vi "GetProperty.vi"(7 "Get":bool, 8 "error in (no error)":errorcluster, 9 "SubIndex":u8 format="%x", 10 "Index":u16 format="%x", 11 "Template SoftMotion Drive Interface Plug-in Class in":refnum<class "Template SoftMotion Drive Interface Plug-in Class.lvclass">) -> (0 "error out":errorcluster, 1 "Data":u32, 2 "Done":bool, 3 "Template SoftMotion Drive Interface Plug-in Class out":refnum<class "Template SoftMotion Drive Interface Plug-in Class.lvclass">)   [LabVIEW 2014, in "Template SoftMotion Drive Interface Plug-in Class.lvclass"]
uses:
  Template SoftMotion Drive Interface Plug-in Class.lvclass
  <vilib>/Motion/plugins/PluginFramework/nismPluginAxisBase/nismPluginAxisBaseClass.lvclass/nismPluginAxisBaseClass.ctl
  <vilib>/Motion/plugins/PluginFramework/nismPluginAxisBase/ReadEtherCATSlaveReference.vi
  <resource>/objmgr/IndComECAT.rc
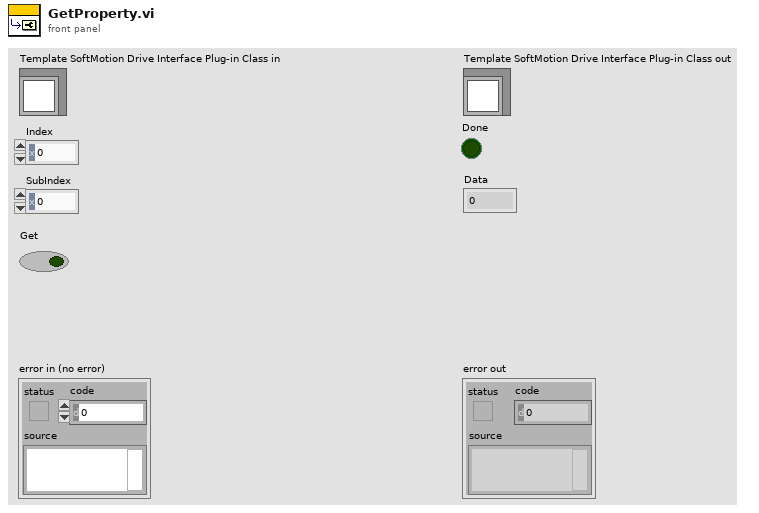
[diagram p1: front panel]
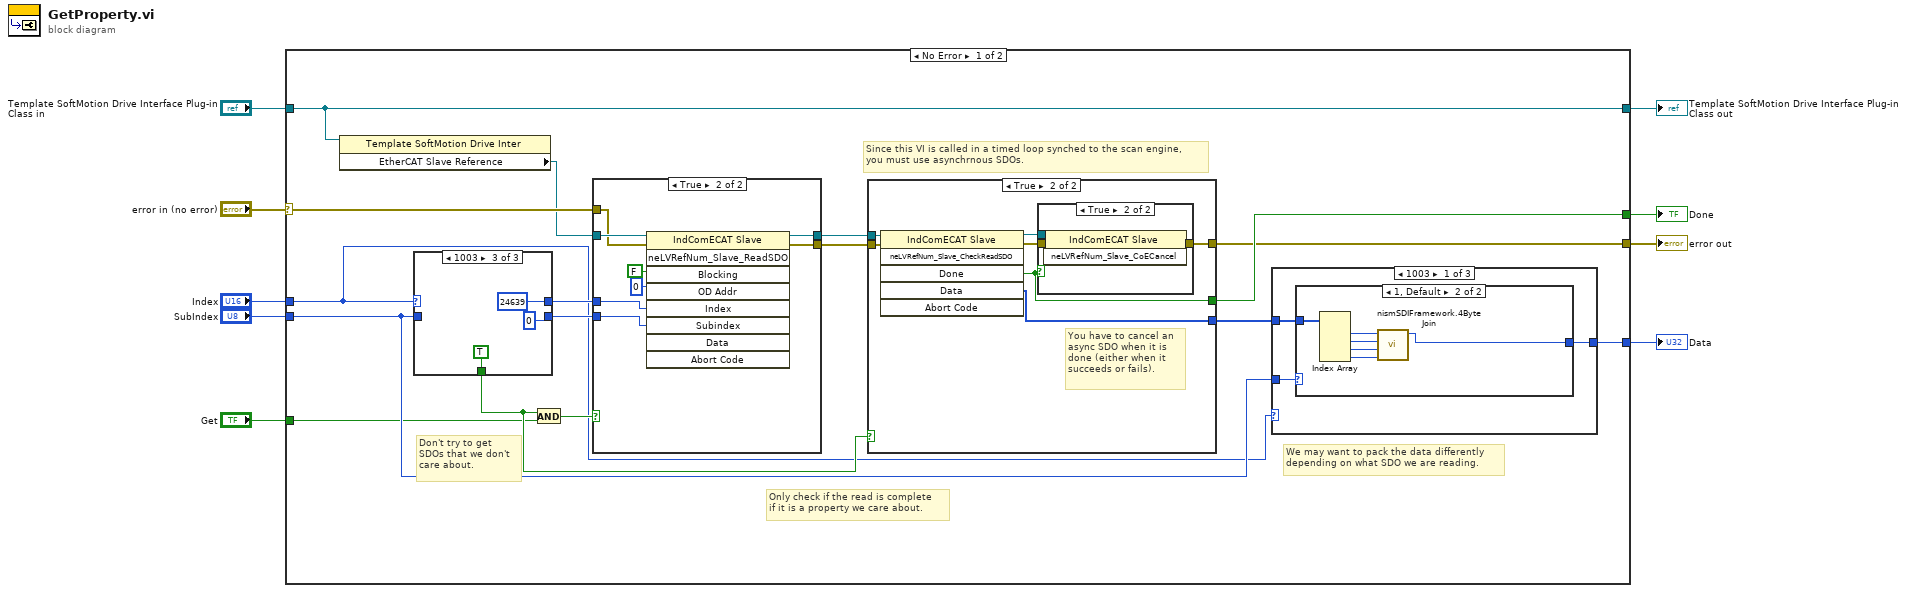
[diagram p0: block diagram]
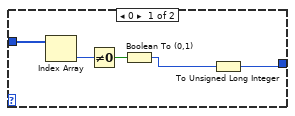
[diagram p2: hidden frame]
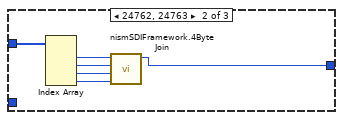
[diagram p3: hidden frame]
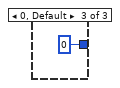
[diagram p4: hidden frame]
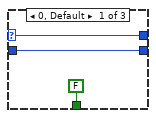
[diagram p5: hidden frame]
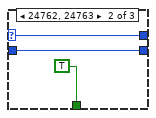
[diagram p6: hidden frame]
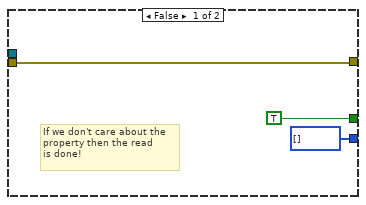
[diagram p7: hidden frame]
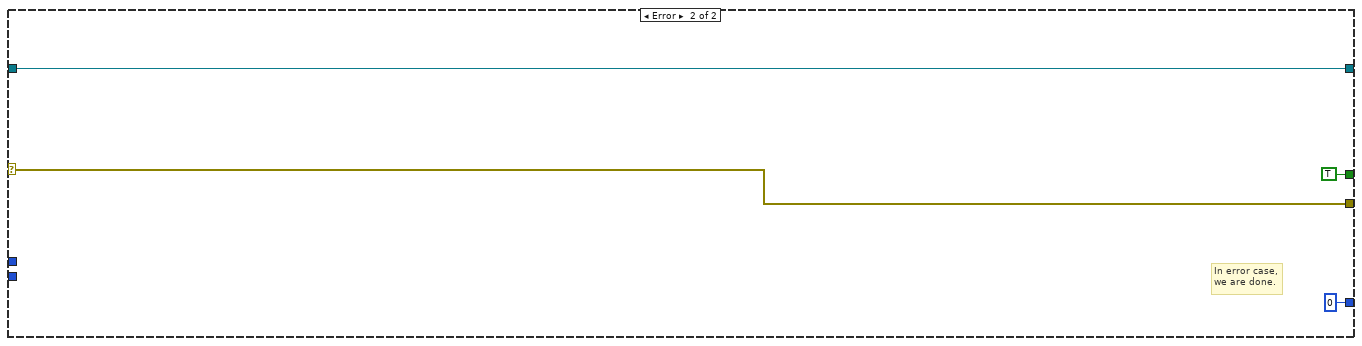
[diagram p10: hidden frame]
diagram:
  n1 = case shown="No Error" "error in (no error)" {
    selector: "error in (no error)" -> [w16 w82]
    tunnel: [w13 w83] -> w4
    tunnel: "Template SoftMotion Drive Interface Plug-in Class in" -> [w13 w83]
    tunnel: "Index" -> [w10 _]
    tunnel: "SubIndex" -> [w20 _]
    tunnel: "Get" -> [w19 _]
    tunnel: [w17 TRUE ("Done")] -> w3
    tunnel: [w15 w82] -> w1
    tunnel: [w14 0] -> w2
    frame No Error {
      # "Since this VI is called in a timed loop synched to the scan engine,\nyou must use asynchrnous SDOs."
      # "We may want to pack the data differently\ndepending on what SDO we are reading."
      # "Don't try to get\nSDOs that we don't\ncare about."
      # "Only check if the read is complete\nif it is a property we care about."
      n2 = property class="Template SoftMotion Drive Inter"(reference=w13) -> ("EtherCAT Slave Reference"=w12:refnum<k21>)  [unwired: 1 in, 2 out]
      n3 = case shown="1003" w10 {
        selector: w10 -> [w48 w50 _]
        tunnel: w20 -> [w49 w51 _]
        tunnel: [FALSE TRUE TRUE] -> w22
        tunnel: [w48 w50 u16 24639 ("Index")] -> w11
        tunnel: [w49 w51 u8 0 ("SubIndex")] -> w18
        frame 0, Default {
        }
        frame 24762, 24763 {
        }
        frame 4099 {
        }
      }
      n4 = And(x=w22, y=w19) -> (x .and. y?=w23:bool)
      n5 = case shown="True" w23 {
        tunnel: w12 -> [w71 w73]
        tunnel: w11 -> [_ w77]
        tunnel: w18 -> [_ w76]
        tunnel: w16 -> [w70 w72]
        tunnel: [w71 w75] -> w25
        tunnel: [w70 w74] -> w24
        frame False {
        }
        frame True {
          n6 = invoke class="IndComECAT Slave" method="neLVRefNum_Slave_ReadSDO"(reference=w73, error in=w72, "Blocking"=FALSE, "OD Addr"=u16 0, "Index"=w77, "Subindex"=w76) -> (reference out=w75:refnum<k21>, error out=w74:errorcluster)  [unwired: 3 in, 7 out]
        }
      }
      n7 = case shown="True" w22 {
        tunnel: w25 -> [_ w65]
        tunnel: w24 -> [w58 w64]
        tunnel: [w58 w61] -> w15
        tunnel: [TRUE ("Done") w60] -> w17
        tunnel: [u8[] [] ("Data") w59] -> w21
        frame False {
          # "If we don't care about the\nproperty then the read\nis done!"
        }
        frame True {
          # "You have to cancel an\nasync SDO when it is \ndone (either when it\nsucceeds or fails)."
          n8 = invoke class="IndComECAT Slave" method="neLVRefNum_Slave_CheckReadSDO"(reference=w65, error in=w64) -> (reference out=w63:refnum<k21>, error out=w62:errorcluster, "Done"=w60:bool, "Data"=w59:u8[])  [unwired: 4 in, 2 out]
          n9 = case shown="True" w60 {
            tunnel: w63 -> [_ w69]
            tunnel: w62 -> [w66 w68]
            tunnel: [w66 w67] -> w61
            frame False {
            }
            frame True {
              n10 = invoke class="IndComECAT Slave" method="neLVRefNum_Slave_CoECancel"(reference=w69, error in=w68) -> (error out=w67:errorcluster)  [unwired: 1 in, 2 out]
            }
          }
        }
      }
      n11 = case shown="1003" w10 {
        tunnel: w21 -> [w28 w45 _]
        tunnel: w20 -> [w27 _ _]
        tunnel: [w26 w40 u32 0] -> w14
        frame 4099 {
          n12 = case shown="1, Default" w27 {
            tunnel: w28 -> [w33 w39]
            tunnel: [w29 w34] -> w26
            frame 0 {
              n13 = Index Array(array=w33) -> (element=w32:u8)  [unwired: 1 in]
              n14 = Not Equal To 0?(x=w32) -> (x != 0?=w31:bool)
              n15 = Boolean To (0,1)(Boolean=w31) -> (0, 1=w30:i16)
              n16 = To Unsigned Long Integer(number=w30) -> (unsigned 32bit integer=w29:u32)
            }
            frame 1, Default {
              n17 = Index Array(array=w39) -> (element #1=w38:u8, element #2=w37:u8, element #3=w36:u8, element #4=w35:u8)  [unwired: 4 in]
              n18 = call <vilib>:"nismSDIFramework.4ByteJoin.vi"("hihi"=w35, "hilo"=w36, "lohi"=w37, "lolo"=w38) -> ("4 byte out"=w34:u32)  [unwired: 7 in]
            }
          }
        }
        frame 24762, 24763 {
          n19 = Index Array(array=w45) -> (element #1=w44:u8, element #2=w43:u8, element #3=w42:u8, element #4=w41:u8)  [unwired: 4 in]
          n20 = call <vilib>:"nismSDIFramework.4ByteJoin.vi"("hihi"=w41, "hilo"=w42, "lohi"=w43, "lolo"=w44) -> ("4 byte out"=w40:u32)  [unwired: 7 in]
        }
        frame 0, Default {
        }
      }
    }
    frame Error {
      # "In error case,\nwe are done."
    }
  }
  "error out" <- w1
  "Template SoftMotion Drive Interface Plug-in Class out" <- w4
  "Data" <- w2
  "Done" <- w3
